vi "CODMn通讯.vi"() -> ()   [LabVIEW 2016, in "斯坦道CODMn.lvlib"]
uses:
  <vilib>/NI/Modbus Library/API/Wrapper/Create TCP Slave.vi
  <vilib>/NI/Modbus Library/API/slave/Modbus Slave.lvclass
  <vilib>/Plasmionique/MB Master/MB_Master/MB_Master.lvclass
  <vilib>/Plasmionique/MB Master/MB Master.lvlib
  <vilib>/Utility/config.llb/NI_LVConfig.lvlib
  <vilib>/NI/Modbus Library/API/Wrapper/API Main.lvlib
panel:
  in  "读取数据":bool
  in  "释放串口":bool
  in  "打开串口":bool
  out "队列中元素数量":i32
  out "元素":cluster{"命令":string}[](array[cluster])
  out "待处理插入数量":i32
  out "读取公式":u16[](array[numeric])
  out "读取参数":u16[](array[numeric])
  out "数据存储":u16[](array[numeric])
  out "温度":bool[](array[boolean])
  out "M输出点":bool[](array[boolean])
  out "ORP、时间":u16[](array[numeric])
  out "测量状态":u16[](array[numeric])
  out "通讯状态":bool
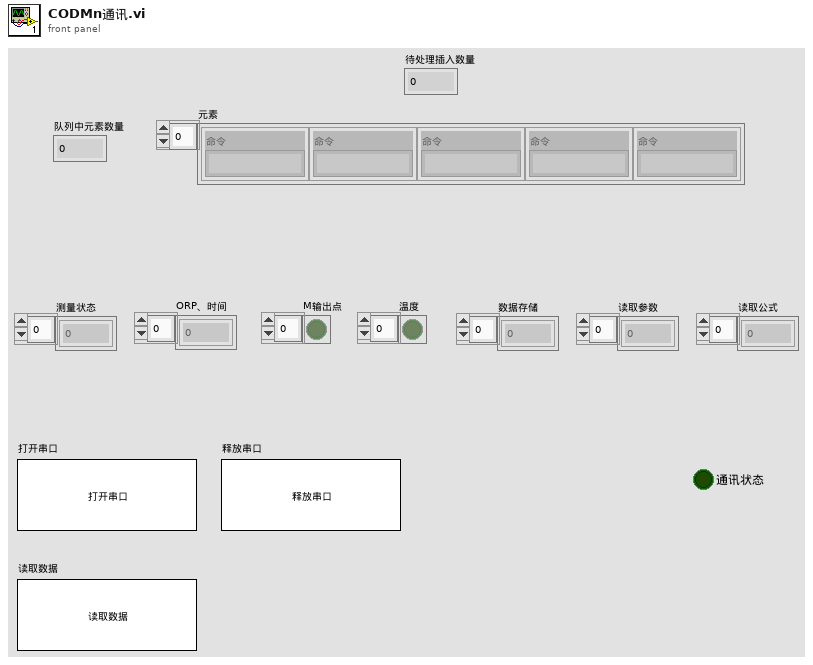
[diagram p1: front panel]
types:
  T1 = cluster{"测量模式":enum16{"水样测量", "标样核查", "零点核查", "跨度核查", "空白测试", "加标回收", "平行样", "校零", "校标"}}
  T2 = cluster{"命令":string, "测量模式":enum16{"水样测量", "标样核查", "零点核查", "跨度核查", "空白测试", "加标回收", "平行样", "校零", "校标"}, "CODMn量程切换":enum32{"H", "L", "AUTO"}}
  T3 = typedef "NI_LVConfig.lvlib/Config Data RefNum.ctl" = refnum<k1>
  T4 = enum16{"空闲", "水样测试", "标样核查", "零点核查", "跨度核查", "空白测试", "平行样测试", "质控样", "空白校准", "标样校准", "加标回收"}
  T5 = enum16{"水样测量", "标样核查", "零点核查", "跨度核查", "空白测试", "加标回收", "平行样", "校零", "校标"}
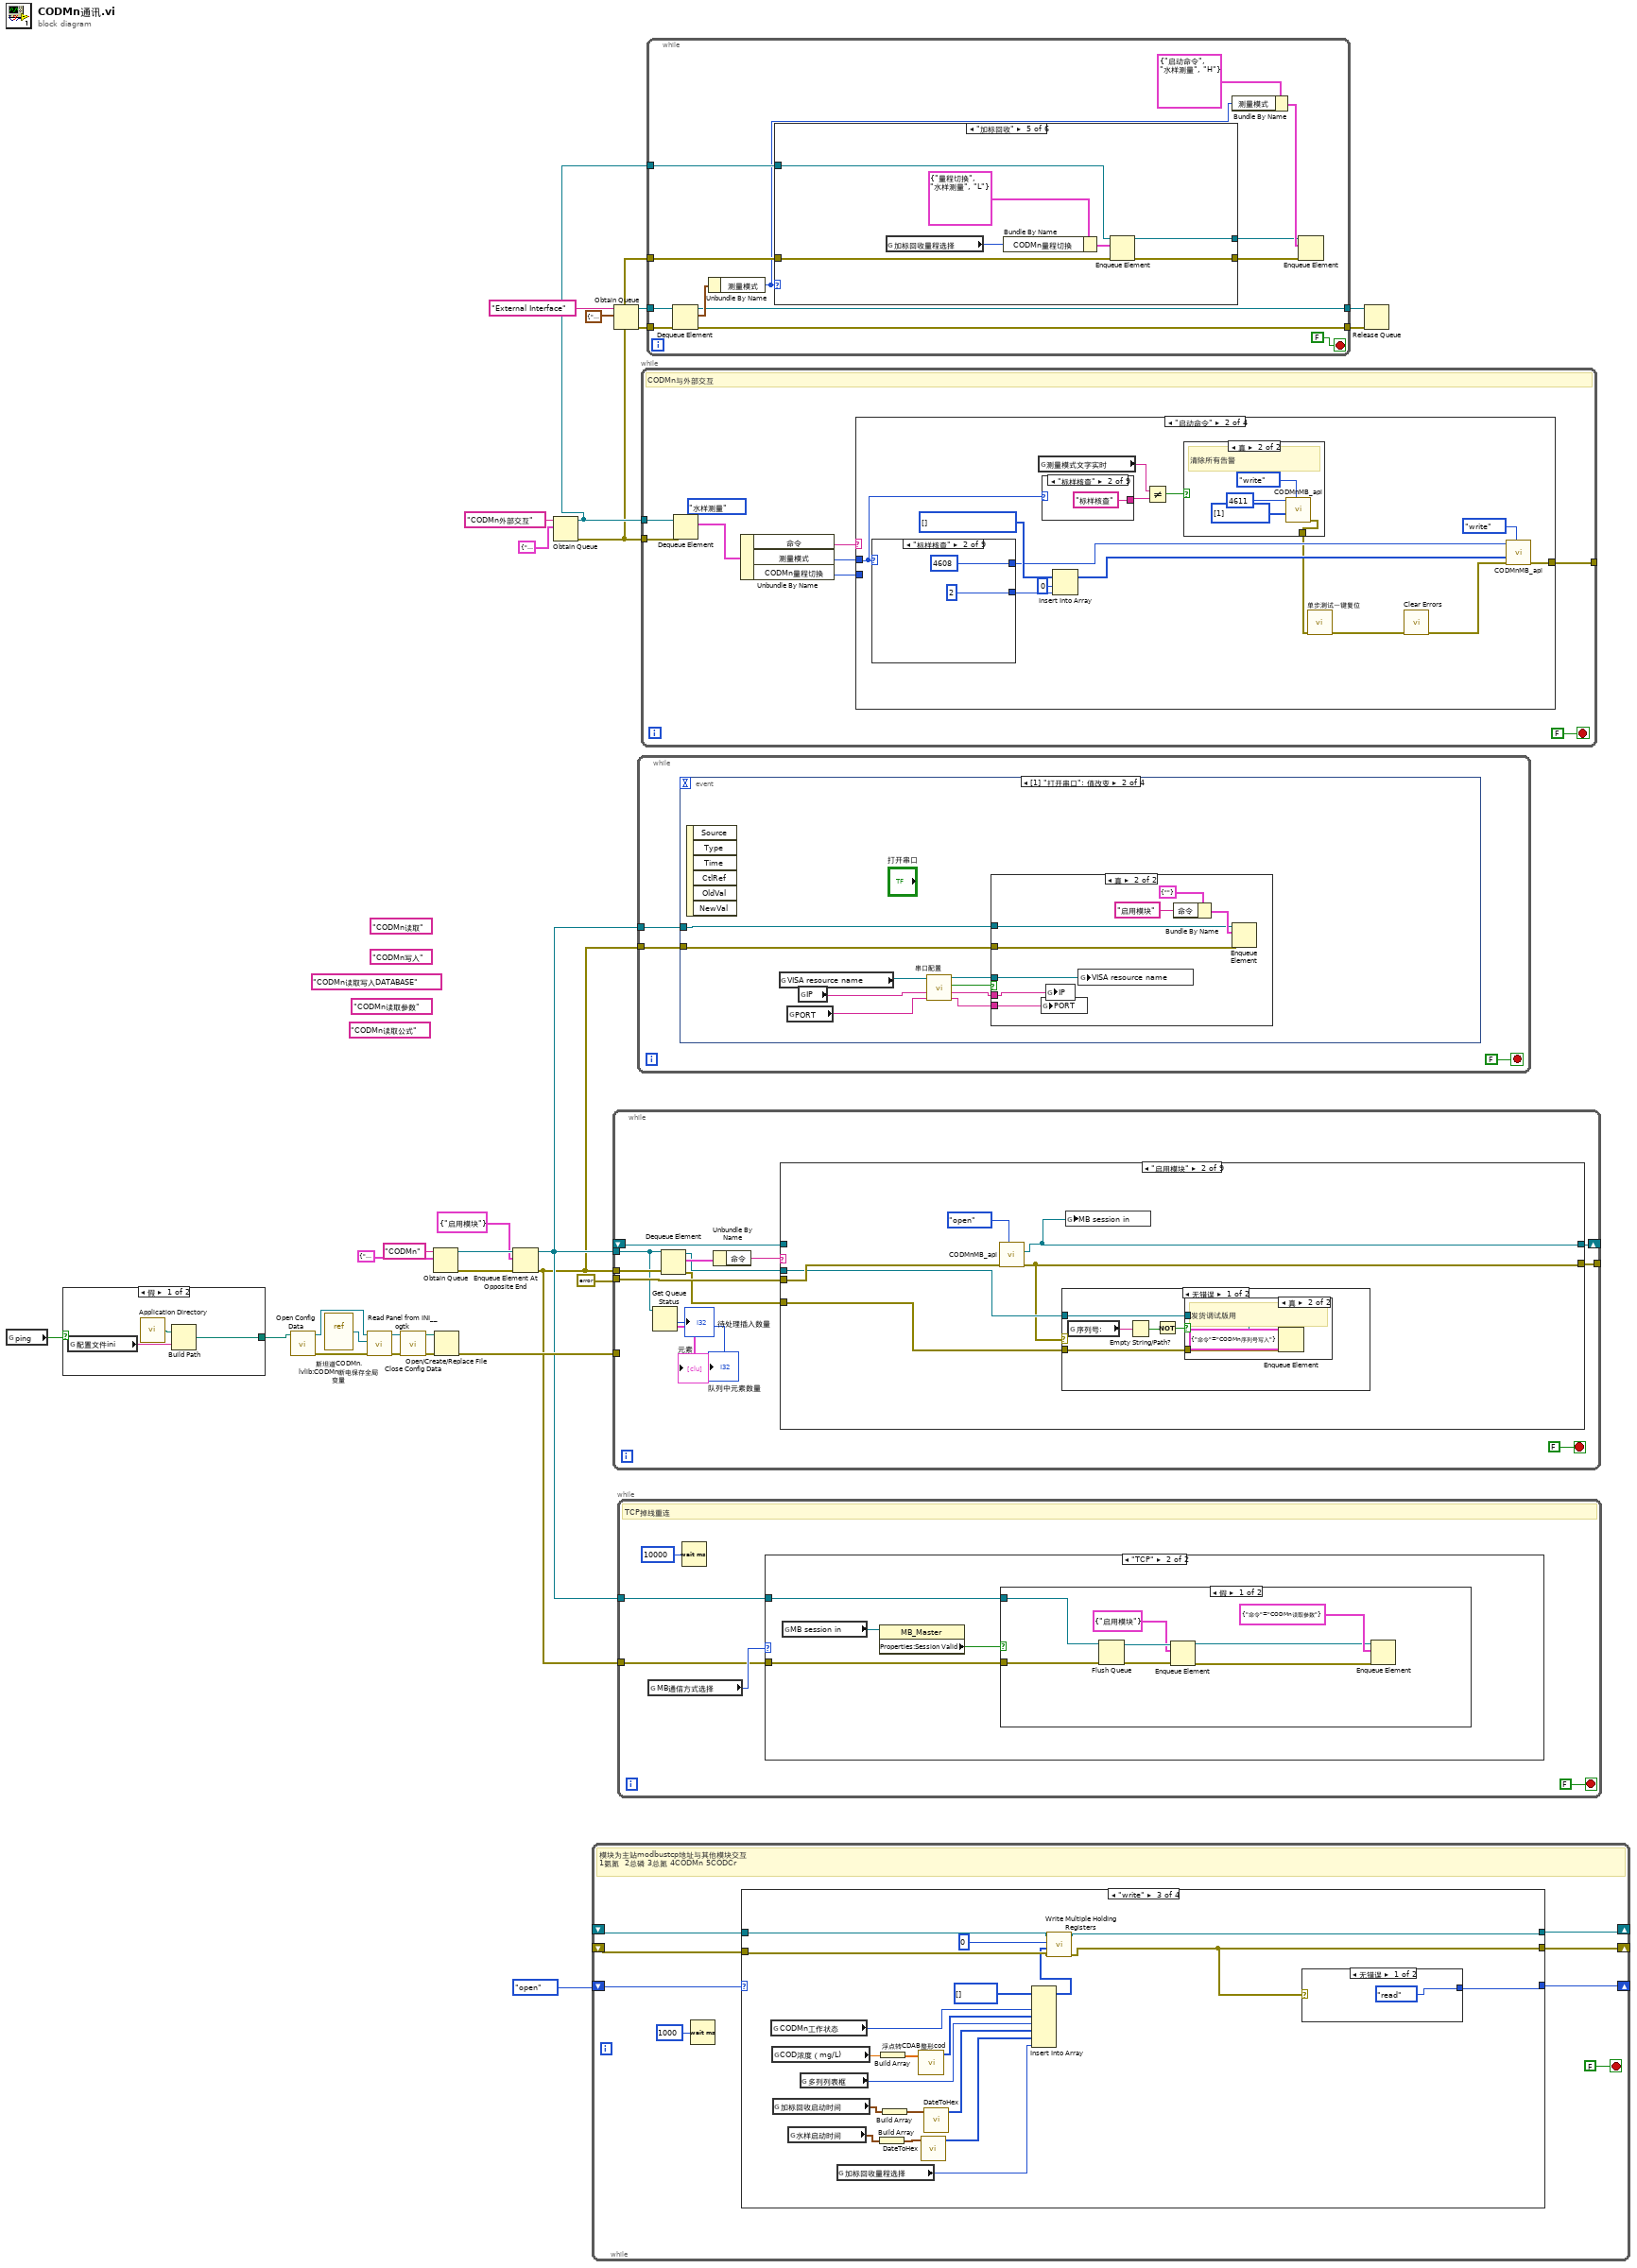
[diagram p0: block diagram]
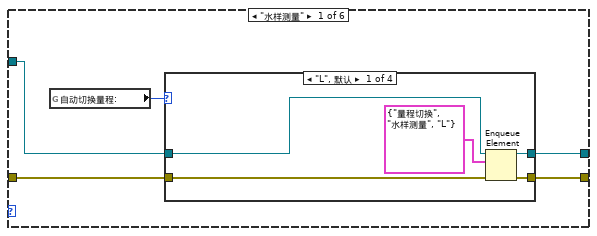
[diagram p2: hidden frame]
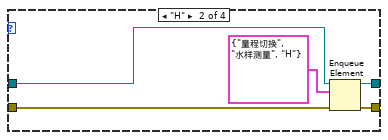
[diagram p3: hidden frame]
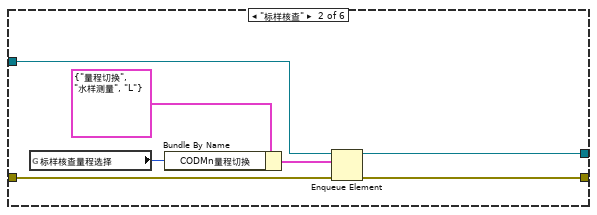
[diagram p6: hidden frame]
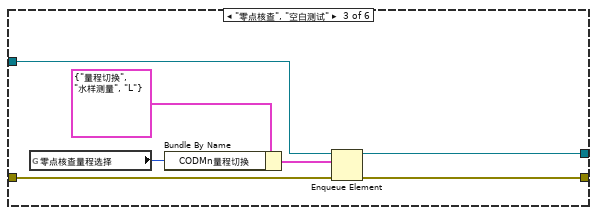
[diagram p7: hidden frame]
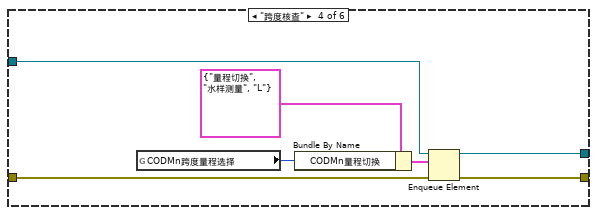
[diagram p8: hidden frame]
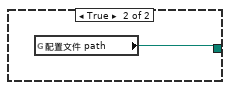
[diagram p10: hidden frame]
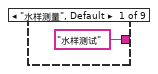
[diagram p13: hidden frame]
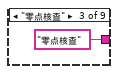
[diagram p14: hidden frame]
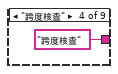
[diagram p15: hidden frame]
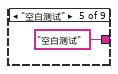
[diagram p16: hidden frame]
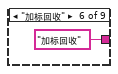
[diagram p17: hidden frame]
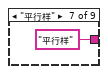
[diagram p18: hidden frame]
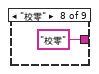
[diagram p19: hidden frame]
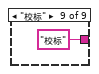
[diagram p20: hidden frame]
diagram:
  (unwired) "CODMn读取公式" ("名称（未命名）")
  (unwired) "CODMn读取写入DATABASE" ("名称（未命名）")
  (unwired) "CODMn读取参数" ("名称（未命名）")
  (unwired) "CODMn读取" ("名称（未命名）")
  (unwired) "CODMn写入" ("名称（未命名）")
  n1 = global read "CODMN外部API.vi" "ping"() -> (w10:bool)
  n2 = case shown="假" w10 {
    tunnel: [w30 w33] -> w9
    frame False {
      n3 = global read "COD内部交互全局.vi" "配置文件ini"() -> (w32:string)
      n4 = call <vilib>:"Application Directory.vi"() -> ("Application Directory"=w31:path)
      n5 = Build Path(base path=w31, name or relative path=w32) -> (appended path=w30:path)
    }
    frame True {
      n6 = global read "CODMN外部API.vi" "配置文件 path"() -> (w33:path)
    }
  }
  n7 = call <vilib>:"Open Config Data.vi"("configuration file path"=w9) -> ("error out"=w20:errorcluster, "refnum"=w23:T3)  [unwired: 8 in, 1 out]
  n8 = vi-ref "斯坦道CODMn.lvlib:CODMn断电保存全局变量.vi"() -> (w22:refnum<vi>)
  n9 = call <userlib>:"Read Panel from INI__ogtk.vi"("error in (no error)"=w20, "VI ref"=w22, "refnum"=w23) -> ("error out"=w19:errorcluster, "refnum out"=w21:T3)  [unwired: 7 in]
  n10 = call <vilib>:"Close Config Data.vi"("error in (no error)"=w19, "refnum"=w21) -> ("error out"=w18:errorcluster, "file path"=w17:path)  [unwired: 8 in]
  n11 = Obtain Queue(name (unnamed)="CODMn" ("名称（未命名）"), element data type=cluster{"命令":string} {"命令"="启用模块"} ("元素")) -> (queue out=w26:refnum<queue>, error out=w25:errorcluster)  [unwired: 3 in, 1 out]
  n12 = Open/Create/Replace File(file path (use dialog)=w17, error in=w18) -> (error out=w16:errorcluster)  [unwired: 4 in, 2 out]
  n13 = Enqueue Element At Opposite End(queue=w26, element=cluster{"命令":string} {"命令"="启用模块"} ("元素"), error in (no error)=w25) -> (queue out=w14:refnum<queue>, error out=w13:errorcluster)  [unwired: 1 in, 1 out]
  n14 = Obtain Queue(name (unnamed)="CODMn外部交互" ("名称（未命名）"), element data type=T2 {"命令"="启动命令", "测量模式"=enum."水样测量", "CODMn量程切换"=enum."AUTO"} ("元素")) -> (queue out=w4:refnum<queue>, error out=w3:errorcluster)  [unwired: 3 in, 1 out]
  n15 = while {
    shift-right: [w39] -> _
    shift-left: _ -> [w41]
    shift-right: [w38] -> _
    shift-left: _ -> [w40]
    shift-right: [w35] -> _
    shift-left: enum16{"open", "read", "write", "close"}."open" -> [w36]
    stop <- FALSE stop-if-true
    # "模块为主站modbustcp地址与其他模块交互\n1氨氮  2总磷 3总氮 4CODMn 5CODCr"
    n16 = Wait (ms)(milliseconds to wait=u32 1000 ("等待时间（毫秒）")) -> ()  [unwired: 1 out]
    n17 = case shown="\"write\"" w36 {
      selector: w36 -> [w50 _ _ _]
      tunnel: w41 -> [w44 w58 w82 w88]
      tunnel: w40 -> [w43 w57 w79 w87]
      tunnel: [w47 w53 w81 w88] -> w39
      tunnel: [w46 w54 w80 w90] -> w38
      tunnel: [w49 w61 w83 enum16{"open", "read", "write", "close"}."open"] -> w35
      frame "open", Default {
        n18 = call-dynamic "Shutdown.vi"("error in"=w43, "Modbus slave in"=w44) -> ("error out"=w42:errorcluster)  [unwired: 9 in]
        n19 = call <vilib>:"Clear Errors.vi"("error in (no error)"=w42) -> ("error out"=w45:errorcluster)  [unwired: 5 in, 1 out]
        n20 = call-poly <vilib>:"Create Modbus Instance.vi"("error in"=w45, "port (502)"=u16 4) -> ("error out"=w46:errorcluster, "TCP slave instance"=w47:refnum<class "Modbus Slave.lvclass">)  [unwired: 8 in]
        n21 = case shown="错误" w46 {
          tunnel: w50 -> [_ w52]
          tunnel: [enum16{"open", "read", "write", "close"}."write" w52] -> w49
          frame No Error {
          }
          frame Error {
          }
        }
      }
      frame "read" {
        n22 = call-dynamic <vilib>:"Read Holding Registers.vi"("error in"=w57, "number of inputs"=u16 1, "starting address"=u16 257, "Modbus slave in"=w58) -> ("error out"=w54:errorcluster, "register values"=w56:u16[], "Modbus slave out"=w53:refnum<class "Modbus Slave.lvclass">)  [unwired: 5 in]
        n23 = Index Array(array=w56) -> (element=w55:u16)  [unwired: 1 in]
        n24 = global write "CODMN外部API.vi" "CODMn状态"(w55) -> ()
        n25 = case shown="无错误" w54 {
          tunnel: [enum16{"open", "read", "write", "close"}."write" enum16{"open", "read", "write", "close"}."close"] -> w61
          frame No Error {
          }
          frame Error {
          }
        }
      }
      frame "write" {
        n26 = global read "COD测量模式全局.vi" "CODMn工作状态"() -> (w69:T4)
        n27 = global read "COD浓度全局变量.vi" "COD浓度（mg/L)"() -> (w71:dbl)
        n28 = global read "COD测量模式全局.vi" "加标回收启动时间"() -> (w74:timestamp)
        n29 = global read "COD测量模式全局.vi" "水样启动时间"() -> (w76:timestamp)
        n30 = global read "运行时序全局变量.vi" "多列列表框"() -> (w73:i32)
        n31 = global read "CODMn断电保存全局变量.vi" "加标回收量程选择"() -> (w64:enum32{"H", "L", "AUTO"})
        n32 = Build Array(w76) -> (w75:timestamp[])
        n33 = Build Array(w71) -> (w70:dbl[])
        n34 = Build Array(w74) -> (w67:timestamp[])
        n35 = call "浮点转CDAB整形cod.vi"("浮点数"=w70) -> ("CDAB整形输出"=w72:u16[])  [unwired: 10 in]
        n36 = call "DateToHex.vi"("DATE"=w75) -> ("数组"=w78:u16[])  [unwired: 10 in]
        n37 = call "DateToHex.vi"("DATE"=w67) -> ("数组"=w77:u16[])  [unwired: 10 in]
        n38 = Insert Into Array(array=u16[] [] ("values"), new element #1=w69, new element #2=w72, new element #3=w73, new element #4=w77, new element #5=w78, new element #6=w64) -> (w66:u16[])  [unwired: 1 in]
        n39 = call-dynamic "Write Multiple Holding Registers.vi"("error in"=w79, "registers to write"=w66, "starting address"=u16 0, "Modbus slave in"=w82) -> ("error out"=w80:errorcluster, "Modbus slave out"=w81:refnum<class "Modbus Slave.lvclass">)  [unwired: 6 in]
        n40 = case shown="无错误" w80 {
          tunnel: [enum16{"open", "read", "write", "close"}."read" enum16{"open", "read", "write", "close"}."close"] -> w83
          frame No Error {
          }
          frame Error {
          }
        }
      }
      frame "close" {
        n41 = call-dynamic "Shutdown.vi"("error in"=w87, "Modbus slave in"=w88) -> ("error out"=w86:errorcluster)  [unwired: 9 in]
        n42 = call <vilib>:"Clear Errors.vi"("error in (no error)"=w86) -> ("error out"=w90:errorcluster)  [unwired: 5 in, 1 out]
      }
    }
  }
  n43 = while {
    tunnel: w14 -> [w96]
    tunnel: w13 -> [w103]
    tunnel: [w97] -> _
    shift-right: [w100] -> _
    shift-left: _ -> [w99]
    tunnel: errorcluster {"status"=FALSE, "code"=0, "source"=""} ("error out") -> [w98]
    tunnel: w16 -> [_]
    stop <- FALSE stop-if-true
    n44 = Get Queue Status(queue=w96) -> (# pending insert=→"待处理插入数量":i32, # elements in queue=→"队列中元素数量":i32, elements=→"元素":cluster{"命令":string}[])  [unwired: 2 in, 5 out]
    n45 = Dequeue Element(queue=w96, error in (no error)=w103) -> (queue out=w92:refnum<queue>, element=w102:cluster{"命令":string}, error out=w91:errorcluster)  [unwired: 1 in, 1 out]
    n46 = Unbundle By Name(w102) -> ("命令"=w101:string)
    n47 = case shown="\"启用模块\"" w101 {
      tunnel: [w106 w110 w121 w129 w161 w170 w187 w194 w201] -> w100
      tunnel: [w105 w107 w122 w126 w159 w169 w186 w193 w200] -> w97
      tunnel: w99 -> [w106 _ _ w153 w165 w179 w190 w198 w204]
      tunnel: w98 -> [w105 w111 w123 w152 w162 w178 w189 w197 w202]
      tunnel: w92 -> [_ w109 _ _ _ _ _ _ _]
      tunnel: w91 -> [_ w108 _ _ _ _ _ _ _]
      frame Default {
      }
      frame "启用模块" {
        n48 = call "CODMnMB_api.vi"("STEP"=enum16{"open", "read", "write", "close"}."open", "Error in"=w111) -> ("error out"=w107:errorcluster, "MB session out"=w110:refnum<class "MB_Master.lvclass">)  [unwired: 7 in, 1 out]
        n49 = case shown="无错误" w107 {
          tunnel: w109 -> [w117 _]
          tunnel: w108 -> [w116 _]
          frame No Error {
            n50 = global read "COD内部交互全局.vi" "序列号:"() -> (w115:string)
            n51 = Empty String/Path?(string/path=w115) -> (empty?=w114:bool)
            n52 = Not(x=w114) -> (.not. x?=w113:bool)
            n53 = case shown="真" w113 {
              tunnel: w117 -> [_ w120]
              tunnel: w116 -> [_ w119]
              frame False {
              }
              frame True {
                # "发货调试版用"
                n54 = Enqueue Element(queue=w120, element=cluster{"命令":string} {"命令"="CODMn序列号写入"} ("元素"), error in (no error)=w119) -> ()  [unwired: 1 in, 3 out]
              }
            }
          }
          frame Error {
          }
        }
        n55 = global write "COD浓度全局变量.vi" "MB session in"(w110) -> ()
      }
      frame "停用模块" {
        n56 = call "CODMnMB_api.vi"("STEP"=enum16{"open", "read", "write", "close"}."close", "Error in"=w123) -> ("error out"=w122:errorcluster, "MB session out"=w121:refnum<class "MB_Master.lvclass">)  [unwired: 7 in, 1 out]
      }
      frame "CODMn读取" {
        n57 = call <vilib>:"Read Holding Registers.vi"("error in (no error)"=w152, "quantity"=u16 50 ("number of holding registers"), "starting address"=u16 4224, "MB session in"=w153) -> ("error out"=w143:errorcluster, "Registers"=w149:u16[], "MB session out"=w144:refnum<class "MB_Master.lvclass">)  [unwired: 5 in]
        n58 = case shown="无错误" w143 {
          tunnel: w149 -> [w158 _]
          frame No Error {
            n59 = global write "COD内部交互全局.vi" "测量状态"(w158) -> ()
            "测量状态" <- w158
          }
          frame Error {
          }
        }
        n60 = call <vilib>:"Read Holding Registers.vi"("error in (no error)"=w143, "quantity"=u16 10, "starting address"=u16 4101, "MB session in"=w144) -> ("error out"=w139:errorcluster, "Registers"=w142:u16[], "MB session out"=w141:refnum<class "MB_Master.lvclass">)  [unwired: 5 in]
        n61 = case shown="无错误" w139 {
          tunnel: w142 -> [w157 _]
          frame No Error {
            n62 = global write "COD内部交互全局.vi" "ORP、时间"(w157) -> ()
            "ORP、时间" <- w157
          }
          frame Error {
          }
        }
        n63 = call <vilib>:"Read Coils.vi"("error in (no error)"=w139, "quantity"=u16 11, "starting address"=u16 137, "MB session in"=w141) -> ("error out"=w137:errorcluster, "Coils"=w138:bool[], "MB session out"=w140:refnum<class "MB_Master.lvclass">)  [unwired: 5 in]
        n64 = case shown="无错误" w137 {
          tunnel: w138 -> [w156 _]
          frame No Error {
            n65 = global write "COD内部交互全局.vi" "M输出点"(w156) -> ()
            "M输出点" <- w156
          }
          frame Error {
          }
        }
        n66 = call <vilib>:"Read Coils.vi"("error in (no error)"=w137, "quantity"=u16 1, "starting address"=u16 400, "MB session in"=w140) -> ("error out"=w130:errorcluster, "Coils"=w134:bool[], "MB session out"=w131:refnum<class "MB_Master.lvclass">)  [unwired: 5 in]
        n67 = case shown="无错误" w130 {
          tunnel: w134 -> [w155 _]
          frame No Error {
            n68 = global write "COD内部交互全局.vi" "温度"(w155) -> ()
            "温度" <- w155
          }
          frame Error {
          }
        }
        n69 = call <vilib>:"Read Coils.vi"("error in (no error)"=w130, "quantity"=u16 20, "starting address"=u16 500, "MB session in"=w131) -> ("error out"=w126:errorcluster, "Coils"=w125:bool[], "MB session out"=w129:refnum<class "MB_Master.lvclass">)  [unwired: 5 in]
        n70 = case shown="无错误" w126 {
          tunnel: w125 -> [w154 _]
          frame No Error {
            n71 = global write "COD内部交互全局.vi" "报警点位"(w154) -> ()
          }
          frame Error {
          }
        }
        n72 = Unbundle By Name(w126) -> ("status"=w133:bool)
        n73 = Not(x=w133) -> (.not. x?=w132:bool)
        "通讯状态" <- w132
        n74 = global write "COD内部交互全局.vi" "通讯状态"(w132) -> ()
      }
      frame "CODMn读取写入DATABASE" {
        n75 = call <vilib>:"Read Holding Registers.vi"("error in (no error)"=w162, "quantity"=u16 10 ("number of holding registers"), "starting address"=u16 4101, "MB session in"=w165) -> ("error out"=w159:errorcluster, "Registers"=w160:u16[], "MB session out"=w161:refnum<class "MB_Master.lvclass">)  [unwired: 5 in]
        n76 = case shown="无错误" w159 {
          tunnel: w160 -> [w167 _]
          frame No Error {
            n77 = global write "COD内部交互全局.vi" "数据存储"(w167) -> ()
            n78 = global write "COD内部交互全局.vi" "读取写入data"(TRUE ("读取参数显示")) -> ()
            "数据存储" <- w167
          }
          frame Error {
          }
        }
      }
      frame "CODMn读取参数" {
        n79 = call <vilib>:"Read Holding Registers.vi"("error in (no error)"=w178, "quantity"=u16 35 ("number of holding registers"), "starting address"=u16 4272, "MB session in"=w179) -> ("error out"=w173:errorcluster, "Registers"=w175:u16[], "MB session out"=w174:refnum<class "MB_Master.lvclass">)  [unwired: 5 in]
        n80 = case shown="无错误" w173 {
          tunnel: w175 -> [w183 _]
          frame No Error {
            n81 = global write "COD内部交互全局.vi" "读取参数"(w183) -> ()
            n82 = global write "COD内部交互全局.vi" "读取参数显示"(TRUE ("读取参数显示")) -> ()
            "读取参数" <- w183
          }
          frame Error {
          }
        }
        n83 = call <vilib>:"Read Holding Registers.vi"("error in (no error)"=w173, "quantity"=u16 4, "starting address"=u16 5596, "MB session in"=w174) -> ("error out"=w169:errorcluster, "Registers"=w168:u16[], "MB session out"=w170:refnum<class "MB_Master.lvclass">)  [unwired: 5 in]
        n84 = case shown="无错误" w169 {
          tunnel: w168 -> [w181 _]
          frame No Error {
            n85 = global write "COD内部交互全局.vi" "读取浮台参数"(w181) -> ()
            n86 = global write "COD内部交互全局.vi" "读取浮台参数显示"(TRUE ("读取参数显示")) -> ()
          }
          frame Error {
          }
        }
      }
      frame "CODMn读取公式" {
        n87 = call <vilib>:"Read Holding Registers.vi"("error in (no error)"=w189, "quantity"=u16 94 ("number of holding registers"), "starting address"=u16 4616, "MB session in"=w190) -> ("error out"=w186:errorcluster, "Registers"=w188:u16[], "MB session out"=w187:refnum<class "MB_Master.lvclass">)  [unwired: 5 in]
        n88 = case shown="无错误" w186 {
          tunnel: w188 -> [w192 _]
          frame No Error {
            n89 = global write "COD内部交互全局.vi" "读取公式"(w192) -> ()
            n90 = global write "COD内部交互全局.vi" "读取公式显示"(TRUE ("读取参数显示")) -> ()
            "读取公式" <- w192
          }
          frame Error {
          }
        }
      }
      frame "CODMn序列号写入" {
        n91 = global read "COD内部交互全局.vi" "序列号:"() -> (w196:string)
        n92 = call "StringToHex.vi"("STRING"=w196) -> ("数组"=w195:u16[])  [unwired: 10 in]
        n93 = call <vilib>:"Write Multiple Registers.vi"("error in (no error)"=w197, "values"=w195, "starting address"=u16 4298, "MB session in"=w198) -> ("error out"=w193:errorcluster, "MB session out"=w194:refnum<class "MB_Master.lvclass">)  [unwired: 6 in]
      }
      frame "CODMn程序更新" {
        n94 = call <vilib>:"Write Multiple Registers.vi"("error in (no error)"=w202, "values"=u16[] [0], "starting address"=u16 4296, "MB session in"=w204) -> ("error out"=w200:errorcluster, "MB session out"=w201:refnum<class "MB_Master.lvclass">)  [unwired: 6 in]
      }
    }
  }
  n95 = Obtain Queue(name (unnamed)="External Interface" ("名称（未命名）"), element data type=T1 {"测量模式"=enum."水样测量"} ("启动测量模式")) -> (queue out=w6:refnum<queue>, error out=w5:errorcluster)  [unwired: 3 in, 1 out]
  n96 = while "While循环" {
    tunnel: w14 -> [w207]
    tunnel: w13 -> [w206]
    stop <- FALSE stop-if-true
    # "TCP掉线重连"
    n97 = global read "CODMn断电保存全局变量.vi" "MB通信方式选择"() -> (w208:enum16{"串口", "TCP"})
    n98 = Wait (ms)(milliseconds to wait=u32 10000 ("等待时间（毫秒）")) -> ()  [unwired: 1 out]
    n99 = case shown="\"TCP\"" w208 {
      tunnel: w207 -> [_ w212]
      tunnel: w206 -> [_ w211]
      frame "串口", Default {
      }
      frame "TCP" {
        n100 = global read "COD浓度全局变量.vi" "MB session in"() -> (w214:refnum<class "MB_Master.lvclass">)
        n101 = property class="MB_Master"(reference=w214) -> ("Properties:Session Valid"=w213:bool)  [unwired: 1 in, 2 out]
        n102 = case shown="假" w213 {
          tunnel: w212 -> [w219 _]
          tunnel: w211 -> [w218 _]
          frame False {
            n103 = Flush Queue(queue=w219, error in (no error)=w218) -> (queue out=w222:refnum<queue>, error out=w221:errorcluster)  [unwired: 1 out]
            n104 = Enqueue Element(queue=w222, element=cluster{"命令":string} {"命令"="启用模块"} ("元素"), error in (no error)=w221) -> (queue out=w216:refnum<queue>, error out=w215:errorcluster)  [unwired: 1 in, 1 out]
            n105 = Enqueue Element(queue=w216, element=cluster{"命令":string} {"命令"="CODMn读取参数"} ("元素"), error in (no error)=w215) -> ()  [unwired: 1 in, 3 out]
          }
          frame True {
          }
        }
      }
    }
  }
  n106 = while {
    tunnel: w14 -> [w224]
    tunnel: w13 -> [w223]
    stop <- FALSE stop-if-true
    n107 = event shown="[1] \"打开串口\": 值改变" {
      selector: _ -> [_ _ _ _]
      dyn-events: _ -> [_ _ _ _]
      timeout: _ -> [_ _ _ _]
      tunnel: w224 -> [_ w231 w245 w247]
      tunnel: w223 -> [_ w230 w244 w246]
      event Timeout {
        n108 = event-data() -> ()  [unwired: 1 in, 3 out]
      }
      event "打开串口": Value Change {
        n109 = event-data() -> ()  [unwired: 1 in, 6 out]
        n110 = global read "CODMn断电保存全局变量.vi" "VISA resource name"() -> (w234:refnum<visa-resource-name>)
        n111 = global read "CODMn断电保存全局变量.vi" "PORT"() -> (w226:string)
        n112 = global read "CODMn断电保存全局变量.vi" "IP"() -> (w227:string)
        n113 = call "串口配置.vi"("PORT"=w226, "IP"=w227, "请选择串口:"=w234) -> ("PORT 2"=w228:string, "IP 2"=w229:string, "确认 2"=w232:bool, "VISA资源名称 2"=w233:refnum<visa-resource-name>)  [unwired: 4 in, 1 out]
        n114 = case shown="真" w232 {
          tunnel: w233 -> [_ w242]
          tunnel: w231 -> [_ w238]
          tunnel: w230 -> [_ w237]
          tunnel: w229 -> [_ w236]
          tunnel: w228 -> [_ w235]
          frame False {
          }
          frame True {
            n115 = global write "CODMn断电保存全局变量.vi" "PORT"(w235) -> ()
            n116 = global write "CODMn断电保存全局变量.vi" "IP"(w236) -> ()
            n117 = global write "CODMn断电保存全局变量.vi" "VISA resource name"(w242) -> ()
            n118 = Bundle By Name(cluster=cluster{"命令":string} {"命令"=""} ("元素"), "命令"="启用模块" ("名称（未命名）")) -> (w239:cluster{"命令":string})
            n119 = Enqueue Element(queue=w238, element=w239, error in (no error)=w237) -> ()  [unwired: 1 in, 3 out]
          }
        }
      }
      event "释放串口": Value Change {
        n120 = event-data() -> ()  [unwired: 1 in, 6 out]
        n121 = Enqueue Element(queue=w245, element=cluster{"命令":string} {"命令"="停用模块"} ("元素"), error in (no error)=w244) -> ()  [unwired: 1 in, 3 out]
      }
      event "读取数据": Value Change {
        n122 = event-data() -> ()  [unwired: 1 in, 6 out]
        n123 = Enqueue Element(queue=w247, element=cluster{"命令":string} {"命令"="CODMn读取"} ("元素"), error in (no error)=w246) -> ()  [unwired: 1 in, 3 out]
      }
    }
  }
  n124 = while {
    tunnel: w4 -> [w254]
    tunnel: w3 -> [w253]
    tunnel: [w249] -> _
    stop <- FALSE stop-if-true
    (unwired) T5."水样测量" ("测量模式")
    # "CODMn与外部交互"
    n125 = Dequeue Element(queue=w254, error in (no error)=w253) -> (element=w255:T2)  [unwired: 1 in, 3 out]
    n126 = Unbundle By Name(w255) -> ("命令"=w252:string, "测量模式"=w251:T5, "CODMn量程切换"=w250:enum32{"H", "L", "AUTO"})
    n127 = case shown="\"启动命令\"" w252 {
      tunnel: w251 -> [_ w259 _ _]
      tunnel: w250 -> [_ _ _ w309]
      tunnel: [_ w264 w304 w308] -> w249
      frame "假", Default {
      }
      frame "启动命令" {
        n128 = case shown="\"标样核查\"" w259 {
          tunnel: [u16 4608 ("address") u16 4608 ("address") u16 4608 ("address") u16 4608 ("address") u16 4608 ("address") u16 4608 ("address") u16 4608 ("address") u16 4608 ("address") u16 4608 ("address")] -> w266
          tunnel: [u16 1 ("address") u16 2 ("address") u16 3 ("address") u16 4 ("address") u16 5 ("address") u16 7 ("address") u16 6 ("address") u16 8 ("address") u16 9 ("address")] -> w270
          frame "水样测量" {
          }
          frame "标样核查" {
          }
          frame "零点核查" {
          }
          frame "跨度核查" {
          }
          frame "空白测试" {
          }
          frame "加标回收" {
          }
          frame "平行样" {
          }
          frame "校零" {
            n129 = global write "CODMN外部API.vi" "远程反控校零CODMn"(TRUE ("远程反控校准CODMn")) -> ()
          }
          frame "校标" {
            n130 = global write "CODMN外部API.vi" "远程反控校准CODMn"(TRUE ("远程反控校准CODMn")) -> ()
          }
        }
        n131 = global read "COD测量模式全局.vi" "测量模式文字实时"() -> (w260:string)
        n132 = case shown="\"标样核查\"" w259 {
          tunnel: ["水样测试" ("测量模式") "标样核查" ("测量模式") "零点核查" ("测量模式") "跨度核查" ("测量模式") "空白测试" ("测量模式") "加标回收" ("测量模式") "平行样" ("测量模式") "校零" ("测量模式") "校标" ("测量模式")] -> w261
          frame "水样测量", Default {
          }
          frame "标样核查" {
          }
          frame "零点核查" {
          }
          frame "跨度核查" {
          }
          frame "空白测试" {
          }
          frame "加标回收" {
          }
          frame "平行样" {
          }
          frame "校零" {
          }
          frame "校标" {
          }
        }
        n133 = Insert Into Array(array=u16[] [] ("values"), index=0 ("索引"), new element=w270) -> (w265:u16[])
        n134 = Not Equal?(x=w260, y=w261) -> (x != y?=w258:bool)
        n135 = case shown="真" w258 {
          tunnel: [_ w271] -> w257
          frame False {
          }
          frame True {
            # "清除所有告警"
            n136 = call "CODMnMB_api.vi"("STEP"=enum16{"open", "read", "write", "close"}."write", "values"=u16[] [1], "starting address"=u16 4611) -> ("error out"=w271:errorcluster)  [unwired: 6 in, 2 out]
          }
        }
        n137 = call "单步测试一键复位.vi"("Error in"=w257) -> ("error out"=w263:errorcluster)  [unwired: 10 in]
        n138 = call <vilib>:"Clear Errors.vi"("error in (no error)"=w263) -> ("error out"=w262:errorcluster)  [unwired: 5 in, 1 out]
        n139 = call "CODMnMB_api.vi"("STEP"=enum16{"open", "read", "write", "close"}."write", "Error in"=w262, "values"=w265, "starting address"=w266) -> ("error out"=w264:errorcluster)  [unwired: 5 in, 2 out]
      }
      frame "停止命令" {
        n140 = call "CODMnMB_api.vi"("STEP"=enum16{"open", "read", "write", "close"}."write", "values"=u16[] [11], "starting address"=u16 4608) -> ("error out"=w304:errorcluster)  [unwired: 6 in, 2 out]
      }
      frame "量程切换" {
        n141 = case shown="\"H\"" w309 {
          tunnel: [u16[] [1] ("values") u16[] [0] ("values") _] -> w312
          frame "H" {
          }
          frame "L" {
          }
          frame "AUTO", Default {
          }
        }
        n142 = call "CODMnMB_api.vi"("STEP"=enum16{"open", "read", "write", "close"}."write", "values"=w312, "starting address"=u16 4276) -> ("error out"=w308:errorcluster)  [unwired: 6 in, 2 out]
      }
    }
  }
  n143 = while {
    tunnel: w6 -> [w327]
    tunnel: w5 -> [w326]
    tunnel: w4 -> [w323]
    tunnel: w3 -> [w322]
    tunnel: [w316] -> w2
    tunnel: [w315] -> w1
    stop <- FALSE stop-if-true
    n144 = Dequeue Element(queue=w327, error in (no error)=w326) -> (queue out=w316:refnum<queue>, element=w324:T1, error out=w315:errorcluster)  [unwired: 1 in, 1 out]
    n145 = Unbundle By Name(w324) -> ("测量模式"=w319:T5)
    n146 = case "条件结构" shown="\"加标回收\"" w319 {
      tunnel: w323 -> [w331 w350 w357 w364 w371 w376]
      tunnel: w322 -> [w329 w349 w356 w363 w370 w375]
      tunnel: [w330 w348 w355 w362 w369 w376] -> w318
      tunnel: [w328 w347 w354 w361 w368 w375] -> w317
      frame "水样测量" {
        n147 = global read "CODMn断电保存全局变量.vi" "自动切换量程:"() -> (w332:enum16{"L", "H", "自动切换测一次", "自动切换测两次"})
        n148 = case shown="\"L\", 默认" w332 {
          tunnel: w331 -> [w336 w342 w343 w346]
          tunnel: [w334 w341 w343 w346] -> w330
          tunnel: w329 -> [w335 w340 w344 w345]
          tunnel: [w333 w339 w344 w345] -> w328
          frame "L", Default {
            n149 = Enqueue Element(queue=w336, element=T2 {"命令"="量程切换", "测量模式"=enum."水样测量", "CODMn量程切换"=enum."L"} ("元素"), error in (no error)=w335) -> (queue out=w334:refnum<queue>, error out=w333:errorcluster)  [unwired: 1 in, 1 out]
          }
          frame "H" {
            n150 = Enqueue Element(queue=w342, element=T2 {"命令"="量程切换", "测量模式"=enum."水样测量", "CODMn量程切换"=enum."H"} ("元素"), error in (no error)=w340) -> (queue out=w341:refnum<queue>, error out=w339:errorcluster)  [unwired: 1 in, 1 out]
          }
          frame "自动切换测一次" {
          }
          frame "自动切换测两次" {
          }
        }
      }
      frame "标样核查" {
        n151 = global read "CODMn断电保存全局变量.vi" "标样核查量程选择"() -> (w352:enum32{"H", "L", "AUTO"})
        n152 = Bundle By Name(cluster=T2 {"命令"="量程切换", "测量模式"=enum."水样测量", "CODMn量程切换"=enum."L"} ("元素"), "CODMn量程切换"=w352) -> (w353:T2)
        n153 = Enqueue Element(queue=w350, element=w353, error in (no error)=w349) -> (queue out=w348:refnum<queue>, error out=w347:errorcluster)  [unwired: 1 in, 1 out]
      }
      frame "零点核查", "空白测试" {
        n154 = global read "CODMn断电保存全局变量.vi" "零点核查量程选择"() -> (w359:enum32{"H", "L", "AUTO"})
        n155 = Bundle By Name(cluster=T2 {"命令"="量程切换", "测量模式"=enum."水样测量", "CODMn量程切换"=enum."L"} ("元素"), "CODMn量程切换"=w359) -> (w358:T2)
        n156 = Enqueue Element(queue=w357, element=w358, error in (no error)=w356) -> (queue out=w355:refnum<queue>, error out=w354:errorcluster)  [unwired: 1 in, 1 out]
      }
      frame "跨度核查" {
        n157 = global read "CODMn断电保存全局变量.vi" "CODMn跨度量程选择"() -> (w366:enum32{"H", "L", "AUTO"})
        n158 = Bundle By Name(cluster=T2 {"命令"="量程切换", "测量模式"=enum."水样测量", "CODMn量程切换"=enum."L"} ("元素"), "CODMn量程切换"=w366) -> (w365:T2)
        n159 = Enqueue Element(queue=w364, element=w365, error in (no error)=w363) -> (queue out=w362:refnum<queue>, error out=w361:errorcluster)  [unwired: 1 in, 1 out]
      }
      frame "加标回收" {
        n160 = global read "CODMn断电保存全局变量.vi" "加标回收量程选择"() -> (w373:enum32{"H", "L", "AUTO"})
        n161 = Bundle By Name(cluster=T2 {"命令"="量程切换", "测量模式"=enum."水样测量", "CODMn量程切换"=enum."L"} ("元素"), "CODMn量程切换"=w373) -> (w372:T2)
        n162 = Enqueue Element(queue=w371, element=w372, error in (no error)=w370) -> (queue out=w369:refnum<queue>, error out=w368:errorcluster)  [unwired: 1 in, 1 out]
      }
      frame Default {
        # "不切换量程"
      }
    }
    n163 = Bundle By Name(cluster=T2 {"命令"="启动命令", "测量模式"=enum."水样测量", "CODMn量程切换"=enum."H"} ("元素"), "测量模式"=w319) -> (w320:T2)
    n164 = Enqueue Element(queue=w318, element=w320, error in (no error)=w317) -> ()  [unwired: 1 in, 3 out]
  }
  n165 = Release Queue(queue=w2, error in (no error)=w1) -> ()  [unwired: 1 in, 3 out]
